vi "IIR Filtering Using Optional Specs.vi"() -> ()   [LabVIEW 2023]
doc: "Demonstrates the use of the optional IIR filter specifications cluster, allowing an alternate method of specifying the order and cutoff frequencies of the various IIR filter topologies (Butterworth, Chebyshev, and so on)."
uses:
  <vilib>/measure/macond.llb/IIR Filter for 1 Chan.vi
  <vilib>/measure/NI_MABase.lvlib
  <vilib>/measure/NI_MAPro.lvlib
panel:
  in  "Tab Control":T1(tab)
  out "Waveform Graph":waveform(dbl)[](graph)
  out "Magnitude response":cluster{"f0":dbl, "df":dbl, "Mag H(w)":dbl[]}(graph)
  out "Filter phase response":cluster{"f0":dbl, "df":dbl, "Phase H(w)":dbl[]}(graph)
  out "order":i32=5
  in  "optional IIR filter specifications":T2={"Lower PB"=59.0, "Upper PB"=61.0, "Lower SB"=55.0, "Upper SB"=65.0, "PB Gain"=-1.0, "SB Gain"=-60.0, "Scale"=TRUE} {"SB Gain" format="%#.6g"; "PB Gain" format="%#.6g"; "Upper SB" format="%#.6g"; "Lower SB" format="%#.6g"; "Upper PB" format="%#.6g"; "Lower PB" format="%#.6g"}
  in  "noise amplitude":dbl(slide)=0.6530612244897959 scale=0.0..2.0
  in  "reset signal":bool
  in  "IIR filter specifications":T3={"Topology"=enum."Butterworth", "Type"=enum."Bandpass", "Order"=-1, "Lower Fc"=100.0, "Upper Fc"=200.0, "PB Ripple"=1.0, "SB Attenuation"=60.0} {"SB Attenuation" format="%#.6g"; "PB Ripple" format="%#.6g"; "Upper Fc" format="%#.6g"; "Lower Fc" format="%#.6g"}
  in  "reset filter":bool
  in  "sampling info":cluster{"Fs":dbl, "#s":dbl}={"Fs"=1000.0, "#s"=100.0} {"#s" step=100.0 format="%#.6g"; "Fs" step=1000.0 format="%#.6g"}
  in  "signal parameters":T4={"signal type"=enum."Sine Wave", "frequency"=60.0} {"frequency" format="%#.6g"}
  in  "Stop":bool
  # "Overview: Demonstrates the use of the \"optional IIR filter specification\" input to the Digital IIR Filter VI.\nRequirements: LabVIEW Full Development System\nInstructions: \n1. Run the VI.\n2. Notice that the Order, Lower Fc, and Upper Fc controls are disabled.\n3. Select the Filter information tab.\n4.  Change the optional IIR filter specification values and notice the effect on the order value.\n5. Click Stop to stop the VI."
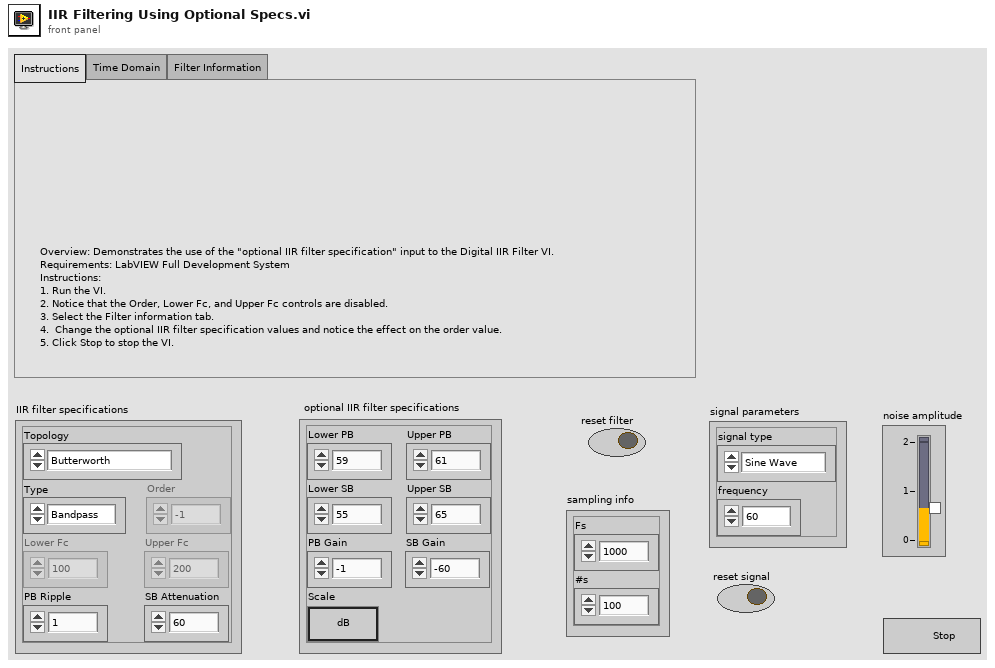
[diagram p1: front panel]
types:
  T1 = enum32{"Instructions", "Time Domain", "Filter Information"}
  T2 = cluster{"Lower PB":dbl, "Upper PB":dbl, "Lower SB":dbl, "Upper SB":dbl, "PB Gain":dbl, "SB Gain":dbl, "Scale":bool}
  T3 = cluster{"Topology":enum16{"Off", "Butterworth", "Chebyshev", "Inverse Chebyshev", "Elliptic", "Bessel"}, "Type":enum16{"Lowpass", "Highpass", "Bandpass", "Bandstop"}, "Order":i32, "Lower Fc":dbl, "Upper Fc":dbl, "PB Ripple":dbl, "SB Attenuation":dbl}
  T4 = cluster{"signal type":enum16{"Sine Wave", "Triangle Wave", "Square Wave", "Sawtooth Wave"}, "frequency":dbl}
  T5 = enum16{"Sine Wave", "Triangle Wave", "Square Wave", "Sawtooth Wave"}
  T6 = cluster{"magnitude H(w)":cluster{"f0":dbl, "df":dbl, "Mag H(w)":dbl[]}, "phase H(w)":cluster{"f0":dbl, "df":dbl, "Phase H(w)":dbl[]}, "order":i32}
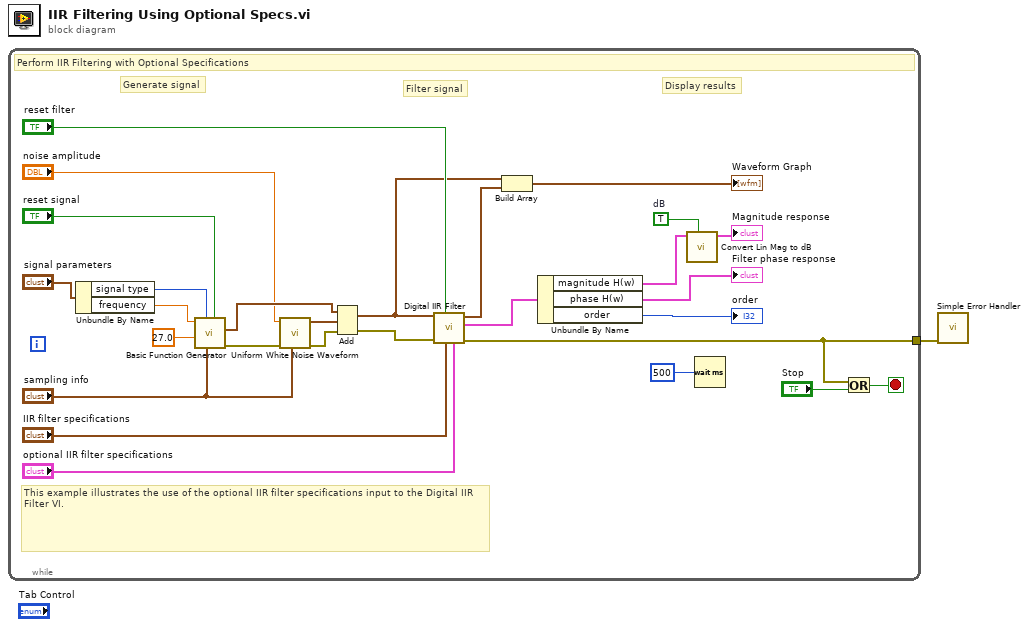
[diagram p0: block diagram]
diagram:
  n1 = while {
    tunnel: [w12] -> w1
    stop <- w28 stop-if-true
    w6 = TRUE  # dB
    # "This example illustrates the use of the optional IIR filter specifications input to the Digital IIR Filter VI."
    # "Display results"
    # "Filter signal"
    # "Generate signal"
    # "Perform IIR Filtering with Optional Specifications"
    n2 = Unbundle By Name("signal parameters") -> ("signal type"=w25:T5, "frequency"=w24:dbl)
    n3 = call <vilib>:"Basic Function Generator.vi"("reset signal"="reset signal", "sampling info"="sampling info", "signal type"=w25, "phase"=27.0, "frequency"=w24) -> ("error out"=w21:errorcluster, "signal out"=w18:waveform(dbl))  [unwired: 4 in, 1 out]
    n4 = call <vilib>:"Uniform White Noise Waveform.vi"("sampling info"="sampling info", "error in (no error)"=w21, "amplitude"="noise amplitude") -> ("error out"=w20:errorcluster, "signal out"=w19:waveform(dbl))  [unwired: 7 in]
    n5 = Add(1:w19, 2:w18, 4:w20) -> (0:w5:waveform(dbl), 3:w14:errorcluster)
    n6 = call-poly <vilib>:"Digital IIR Filter.vi"("optional IIR filter specifications"="optional IIR filter specifications", "IIR filter specifications"="IIR filter specifications", "reset filter"="reset filter", "error in (no error)"=w14, "signal in"=w5) -> ("error out"=w12:errorcluster, "filter information"=w13:T6, "signal out"=w4:waveform(dbl))  [unwired: 4 in]
    n7 = Build Array(w5, w4) -> (→"Waveform Graph":waveform(dbl)[])
    n8 = Unbundle By Name(w13) -> ("magnitude H(w)"=w8:cluster{"f0":dbl, "df":dbl, "Mag H(w)":dbl[]}, "phase H(w)"=→"Filter phase response":cluster{"f0":dbl, "df":dbl, "Phase H(w)":dbl[]}, "order"=→"order":i32)
    n9 = call "Convert Lin Mag to dB.vi"("convert to dB"=w6, "magnitude H(w)"=w8) -> ("magnitude H(w) in dB"=→"Magnitude response":cluster{"f0":dbl, "df":dbl, "Mag H(w)":dbl[]})  [unwired: 9 in]
    n10 = Wait (ms)(milliseconds to wait=u32 500) -> ()  [unwired: 1 out]
    n11 = Or(x=w12, y="Stop") -> (x .or. y?=w28:bool)
  }
  n12 = call <vilib>:"Simple Error Handler.vi"("error in (no error)"=w1) -> ()  [unwired: 4 in, 5 out]
